vi "Request Control Update.vi"(8 "error in (no error)":errorcluster, 11 "Driver in":refnum<class "Driver.lvclass">) -> (0 "error out":errorcluster, 3 "Driver out":refnum<class "Driver.lvclass">)   [LabVIEW 2014, in "Driver.lvlib" / "Driver.lvclass"]
uses:
  Driver.lvclass
  Driver.lvclass/Driver.ctl
  Driver Messages/Get Driver Joystick State Msg/Get Driver Joystick State Msg.lvclass
  <vilib>/ActorFramework/Actor/Actor.lvclass/Actor.ctl
  <vilib>/ActorFramework/Message Enqueuer/Message Enqueuer.lvclass/Message Enqueuer.ctl
  Joystick/Joystick Messages/Request Joystick State Msg/Request Joystick State Msg.lvclass/Request Joystick State Msg.ctl
  <vilib>/ActorFramework/Message Enqueuer/Init from Existing Queue.vi
  <vilib>/ActorFramework/Message Enqueuer/Enqueue.vi
  <vilib>/ActorFramework/Message Priority Queue/Priority Enqueue.vi
  <vilib>/ActorFramework/Message Enqueuer/Message Enqueuer.lvclass
  Joystick/Joystick Messages/Request Joystick State Msg/Request Joystick State Msg.lvclass
  <vilib>/ActorFramework/Actor/Actor.lvclass
  Robot Actor Framework/Utilities/Utilities.lvlib
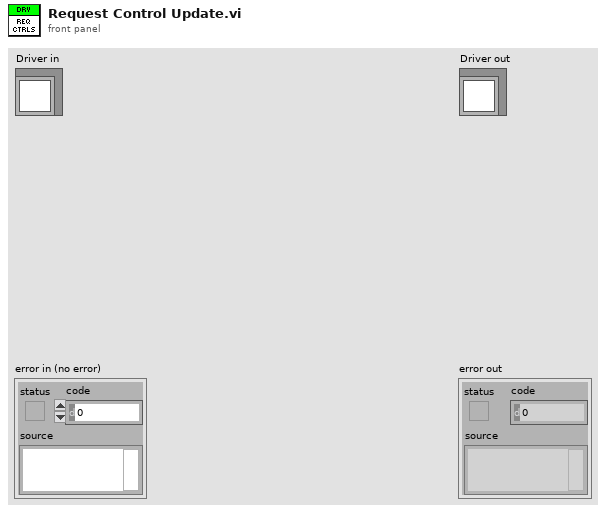
[diagram p1: front panel]
types:
  T1 = enum16{"Critical", "Error", "Warning", "Informational", "Debug"}
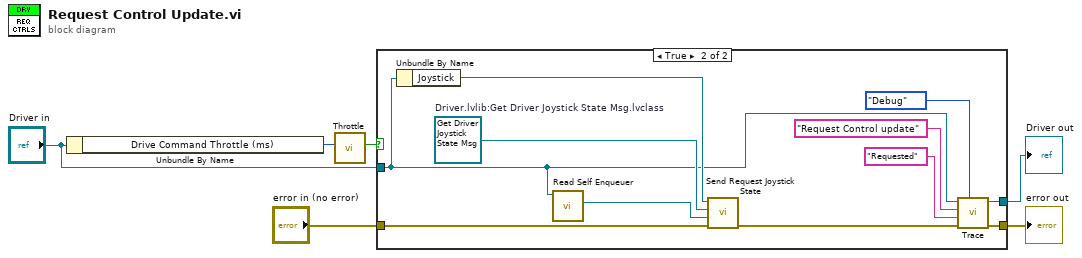
[diagram p0: block diagram]
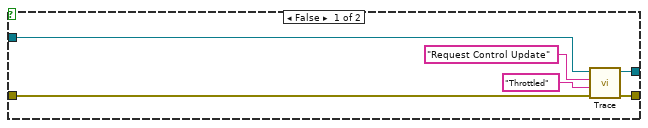
[diagram p2: hidden frame]
diagram:
  n1 = Unbundle By Name("Driver in") -> ("Drive Command Throttle (ms)"=w1:u32)
  n2 = call "Throttle.vi"("Throttle (ms)"=w1) -> ("Past Throttle"=w3:bool)  [unwired: 10 in]
  n3 = case shown="True" w3 {
    tunnel: "error in (no error)" -> [w12 w20]
    tunnel: "Driver in" -> [w10 w19]
    tunnel: [w9 w18] -> w5
    tunnel: [w11 w16] -> w4
    frame False {
      n4 = call-dynamic "Trace.vi"("error in (no error)"=w12, "System Message"="Throttled", "System Action"="Request Control Update", "System Actor in"=w10) -> ("error out"=w11:errorcluster, "System Actor out"=w9:refnum<class "Driver.lvclass">)  [unwired: 6 in]
    }
    frame True {
      w22 = refnum<class "Get Driver Joystick State Msg.lvclass"> refnum  # Driver.lvlib:Get Driver Joystick State Msg.lvclass
      n5 = Unbundle By Name(w19) -> ("Joystick"=w23:refnum<class "Message Enqueuer.lvclass">)
      n6 = call <vilib>:"Read Self Enqueuer.vi"("Actor"=w19) -> ("Self Enqueuer"=w21:refnum<class "Message Enqueuer.lvclass">)  [unwired: 10 in]
      n7 = call "Send Request Joystick State.vi"("error in (no error)"=w20, "Caller Enqueuer"=w21, "Joystick State Msg"=w22, "Message Enqueuer"=w23) -> ("error out"=w17:errorcluster)  [unwired: 6 in, 1 out]
      n8 = call-dynamic "Trace.vi"("Trace Level"=T1."Debug", "error in (no error)"=w17, "System Message"="Requested", "System Action"="Request Control update", "System Actor in"=w19) -> ("error out"=w16:errorcluster, "System Actor out"=w18:refnum<class "Driver.lvclass">)  [unwired: 5 in]
    }
  }
  "error out" <- w4
  "Driver out" <- w5
